vi "sCMOS_acquire_Save_movie.vi"(0 "t0":dbl, 1 "Frames acquired":i32, 4 "N repeat":i32, 5 "error in":errorcluster, 9 "Image IN":T1, 12 "Number of images":i32=10) -> (14 "Stop?":bool, 15 "Frames acquired out":i32, 18 "N repeat out":i32, 19 "error out":errorcluster)   [LabVIEW 2015]
uses:
  <vilib>/vision/Image Controls.llb/IMAQ Image.ctl
  GLOBAL/Global_CAMERA.vi
panel:
  in  "Handle":u32
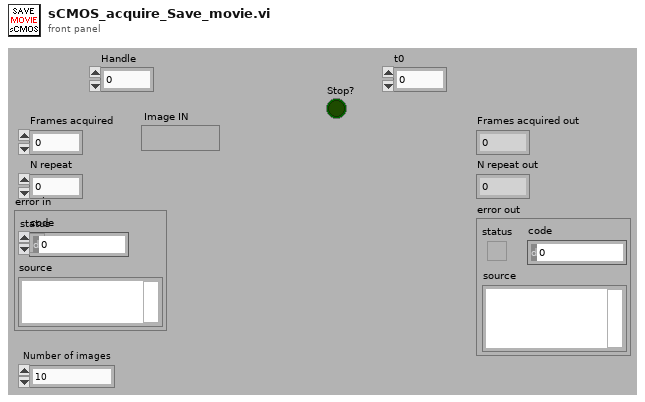
[diagram p1: front panel]
types:
  T1 = typedef "IMAQ Image.ctl" = refnum<image>
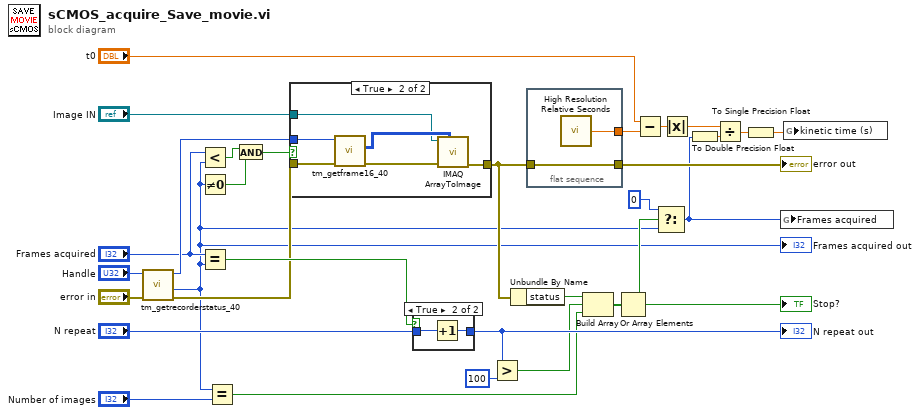
[diagram p0: block diagram]
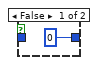
[diagram p3: hidden frame]
diagram:
  n1 = call <userlib>:"tm_getrecorderstatus_40.vi"("error in (no error)"="error in", "Handle"="Handle") -> ("error out"=w17:errorcluster, "Count"=w5:i32, "Handle"=w18:u32)  [unwired: 6 in, 1 out]
  "Frames acquired out" <- w5
  n2 = Less?(x="Frames acquired", y=w5) -> (x < y?=w4:bool)
  n3 = Not Equal To 0?(x=w5) -> (x != 0?=w3:bool)
  n4 = Equal?(x="Frames acquired", y=w5) -> (x = y?=w19:bool)
  n5 = Equal?(x=w5, y="Number of images") -> (x = y?=w25:bool)
  n6 = And(x=w4, y=w3) -> (x .and. y?=w2:bool)
  n7 = case shown="True" w2 {
    tunnel: w18 -> [_ w38]
    tunnel: w17 -> [w32 w37]
    tunnel: "Image IN" -> [_ w34]
    tunnel: [w32 w33] -> w15
    frame False {
    }
    frame True {
      n8 = call <userlib>:"tm_getframe16_40.vi"("error in (no error)"=w37, "Handle in"=w38) -> ("error out"=w35:errorcluster, "Data"=w36:u16[][])  [unwired: 6 in, 2 out]
      n9 = call "IMAQ ArrayToImage"("Image Pixels (U16)"=w36, "error in (no error)"=w35, "Image"=w34) -> ("error out"=w33:errorcluster)  [unwired: 7 in, 1 out]
    }
  }
  n10 = case shown="True" w19 {
    tunnel: "N repeat" -> [_ w41]
    tunnel: [0 w40] -> w29
    frame False {
    }
    frame True {
      n11 = Increment(x=w41) -> (x+1=w40:i32)
    }
  }
  "N repeat out" <- w29
  n12 = Greater?(x=w29, y=100) -> (0:w24:bool)
  n13 = Unbundle By Name(w15) -> ("status"=w23:bool)
  n14 = flat-sequence {
    tunnel: w15 -> [w43]
    tunnel: [w43] -> w14
    tunnel: [w42] -> w13
    frame #0 {
      n15 = call <vilib>:"High Resolution Relative Seconds.vi"() -> ("relative seconds"=w42:dbl)
    }
  }
  n16 = Build Array(w23, w24, w25) -> (w26:bool[])
  n17 = Or Array Elements(Boolean array=w26) -> (logical OR=w22:bool)
  "Stop?" <- w22
  n18 = Subtract(x="t0", y=w13) -> (x-y=w11:dbl)
  n19 = Select(t=0, s=w22, f=w5) -> (s? t:f=w9:i32)
  n20 = Absolute Value(x=w11) -> (abs(x)=w10:dbl)
  n21 = To Double Precision Float(number=w9) -> (double precision float=w7:dbl)
  n22 = Divide(x=w10, y=w7) -> (x/y=w8:dbl)
  n23 = To Single Precision Float(number=w8) -> (single precision float=w1:sgl)
  n24 = global write "Global_CAMERA.vi" "Frames acquired"(w9) -> ()
  n25 = global write "Global_CAMERA.vi" "kinetic time (s)"(w1) -> ()
  "error out" <- w14
